vi "MALT HexStringToByteArray.vi"(3 "String in":string="01234567890") -> (1 "Bytes out":u8[](array[numeric])=[52, 52, 52, 52, 52, 52, 52, 52, 52, 52, 52, 52, 52, 52, 52, 52, 52, 52, 52, 52, 52, 52, 52, 52, 52, 52, 52, 52, 52, 52, 52, 52, 52, 52, 52, 52, 52, 52, 52, 52] format="%02x")   [LabVIEW 2018, in "AltonTech MALT200817.lvlib"]
uses:
  AltonTech MALT200817.lvlib
panel:
  out "length":i32=40
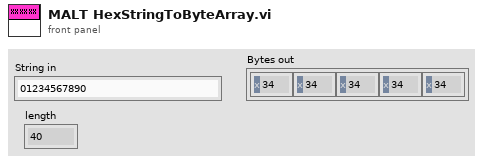
[diagram p1: front panel]
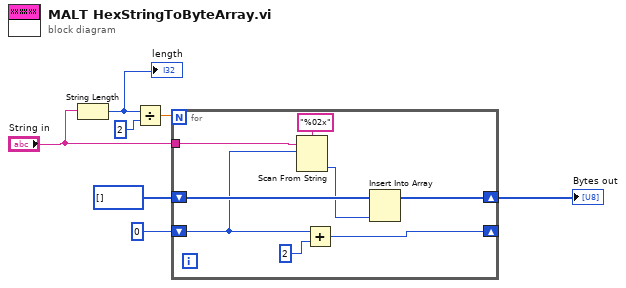
[diagram p0: block diagram]
diagram:
  n1 = String Length(string="String in") -> (length=w3:i32)
  "length" <- w3
  n2 = Divide(x=w3, y=2) -> (x/y=w4:dbl)
  n3 = for {
    N: w4 -> [_]
    tunnel: "String in" -> [w9]
    shift-right: [w13] -> _
    shift-left: 0 ("y") -> [w8]
    shift-right: [w10] -> w1
    shift-left: u8[] [] -> [w12]
    n4 = Scan From String(format string="%02x", input string=w9, initial scan location=w8) -> (output 1=w11:u32)  [unwired: 2 in, 3 out]
    n5 = Add(x=w8, y=2) -> (x+y=w13:i32)
    n6 = Insert Into Array(array=w12, new element=w11) -> (w10:u8[])  [unwired: 1 in]
  }
  "Bytes out" <- w1
